vi "Switch status IO - Human Readable_3voltageamp.vi"(2 "PPMS      DR":bool=TRUE, 3 "Switch status":path=path "C:/LabView/PPMS basic VIs/Switch Status.txt") -> (0 "String":string="I-:2\nV1+:\nI+:1\nV-:5\n")   [LabVIEW 2016, in "pickering.lvclass"]
uses:
  pickering.lvclass
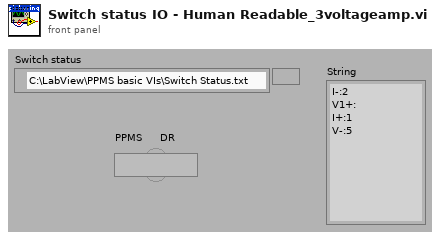
[diagram p1: front panel]
types:
  T1 = typedef "pickering.lvclass/Channels-Array.ctl" = T2[]
  T2 = typedef "pickering.lvclass/Channel-Cluster.ctl" = cluster{"Channel x":T3, "Channel y":T4}
  T3 = typedef "pickering.lvclass/ChannelX-ComboBox.ctl" = string
  T4 = typedef "pickering.lvclass/ChannelY-ComboBox.ctl" = string
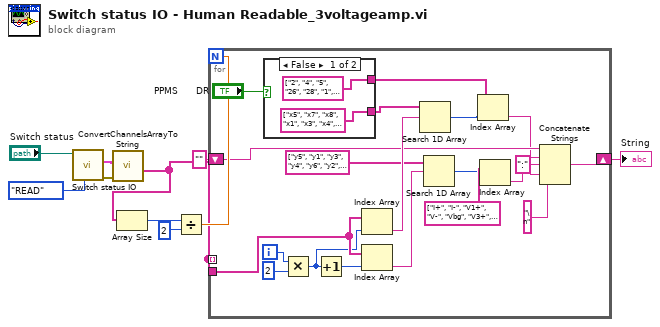
[diagram p0: block diagram]
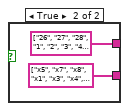
[diagram p2: hidden frame]
diagram:
  n1 = call "Switch status IO.vi"("mode"=enum16{"READ", "WRITE"}."READ", "Path"="Switch status") -> ("error out"=w3:errorcluster, "Channels out"=w2:T1)  [unwired: 7 in, 1 out]
  n2 = call "ConvertChannelsArrayToString.vi"("error in (no error)"=w3, "Channels in"=w2) -> ("String array"=w1:string[])  [unwired: 7 in, 2 out]
  n3 = Array Size(array=w1) -> (size(s)=w6:i32)
  n4 = Divide(x=w6, y=2) -> (x/y=w8:dbl)
  n5 = for {
    N: w8 -> [_]
    tunnel: w1 -> [w30]
    tunnel: w1 -> [_] mode=indexing
    shift-right: [w17] -> w10
    shift-left: "" -> [w16]
    i -> [w28]
    n6 = case shown="False" "PPMS      DR" {
      tunnel: [string[] ["x5", "x7", "x8", "x1", "x3", "x4", "x2", "x6", "x11", "x12", "x10"] string[] ["x5", "x7", "x8", "x1", "x3", "x4", "x2", "x6"]] -> w25
      tunnel: [string[] ["2", "4", "5", "26", "28", "1", "27", "3", "24", "25", "6"] string[] ["26", "27", "28", "1", "2", "3", "4", "5"]] -> w23
      frame False {
      }
      frame True {
      }
    }
    n7 = Multiply(x=w28, y=2) -> (x*y=w26:i32)
    n8 = Increment(x=w26) -> (x+1=w29:i32)
    n9 = Index Array(array=w30, index=w26) -> (element=w24:string)
    n10 = Index Array(array=w30, index=w29) -> (element=w20:string)
    n11 = Search 1D Array(1D array=w25, element=w24) -> (index of element=w22:i32)  [unwired: 1 in]
    n12 = Search 1D Array(1D array=string[] ["y5", "y1", "y3", "y4", "y6", "y2", "y7", "y8"], element=w20) -> (index of element=w18:i32)  [unwired: 1 in]
    n13 = Index Array(array=w23, index=w22) -> (element=w13:string)
    n14 = Index Array(array=string[] ["I+", "I-", "V1+", "V-", "Vbg", "V3+", "V2+", "V2-"], index=w18) -> (element=w15:string)
    n15 = Concatenate Strings(w16, w15, ":" ("string"), w13, "\n" ("string")) -> (w17:string)
  }
  "String" <- w10
